vi "Introduce.vi"(8 "Error In":errorcluster, 11 "Droid in":refnum<class "Droid.lvclass">) -> (0 "Error Out":errorcluster, 3 "Droid out":refnum<class "Droid.lvclass">)   [LabVIEW 2021, in "Droid.lvclass"]
doc: "Show ID of droid in prompt message for user. Comments in Polish."
uses:
  Droid.lvclass
  <vilib>/Utility/error.llb/Error Cluster From Error Code.vi
  <vilib>/ErrorRing/Error Ring.xnode
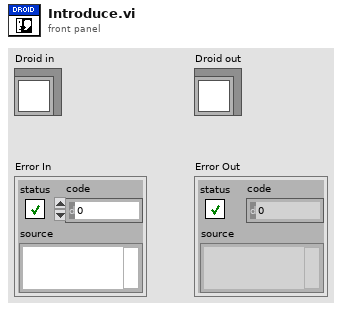
[diagram p1: front panel]
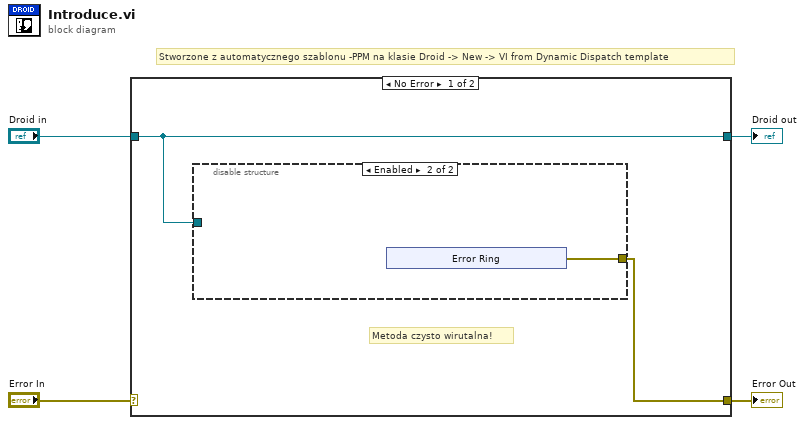
[diagram p0: block diagram]
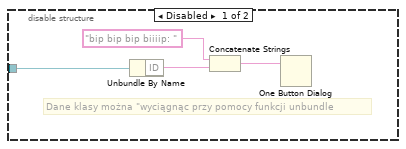
[diagram p2: hidden frame]
diagram:
  # "Stworzone z automatycznego szablonu -PPM na klasie Droid -> New -> VI from Dynamic Dispatch template"
  n1 = case shown="No Error" "Error In" {
    selector: "Error In" -> [_ w18]
    tunnel: [w5 w18] -> w3
    tunnel: [w6 w17] -> w1
    tunnel: "Droid in" -> [w6 w17]
    frame No Error {
      # "Metoda czysto wirutalna!"
      n2 = disable-structure shown="Enabled" {
        disable-tunnel: w6 -> [w10 _]
        disable-tunnel: [_ w11] -> w5
        frame Disabled {
          # "Dane klasy można \"wyciągnąc przy pomocy funkcji unbundle"
          n3 = Unbundle By Name(w10) -> ("ID"=w9:string)
          n4 = Concatenate Strings("bip bip bip biiiip: ", w9) -> (w7:string)
          n5 = One Button Dialog(message=w7) -> ()  [unwired: 1 in, 1 out]
        }
        frame Enabled {
          n6 = xnode "Error Ring"() -> ("error out"=w11:errorcluster)
        }
      }
    }
    frame Error {
    }
  }
  "Error Out" <- w3
  "Droid out" <- w1
